vi "Scripting_GetStateMachineReferences_BaseReference.vi"(0 "Diagram":refnum<vi>, 1 "WhileLoop(False)":bool, 5 "error in (no error)":errorcluster) -> (12 "OutSideWhileLoopDiagram":refnum<vi>, 14 "StateMachine-WhileLoopDiagram":refnum<vi>, 15 "StateMachine-CaseSelector":refnum<vi>, 16 "Found":bool, 17 "Selector.Outside Terminal":refnum<vi>, 19 "error out":errorcluster)   [LabVIEW 2014]
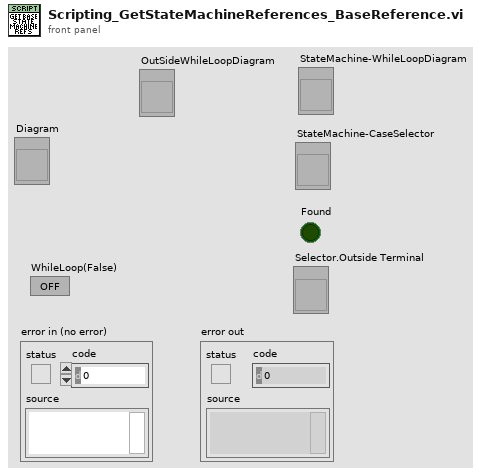
[diagram p1: front panel]
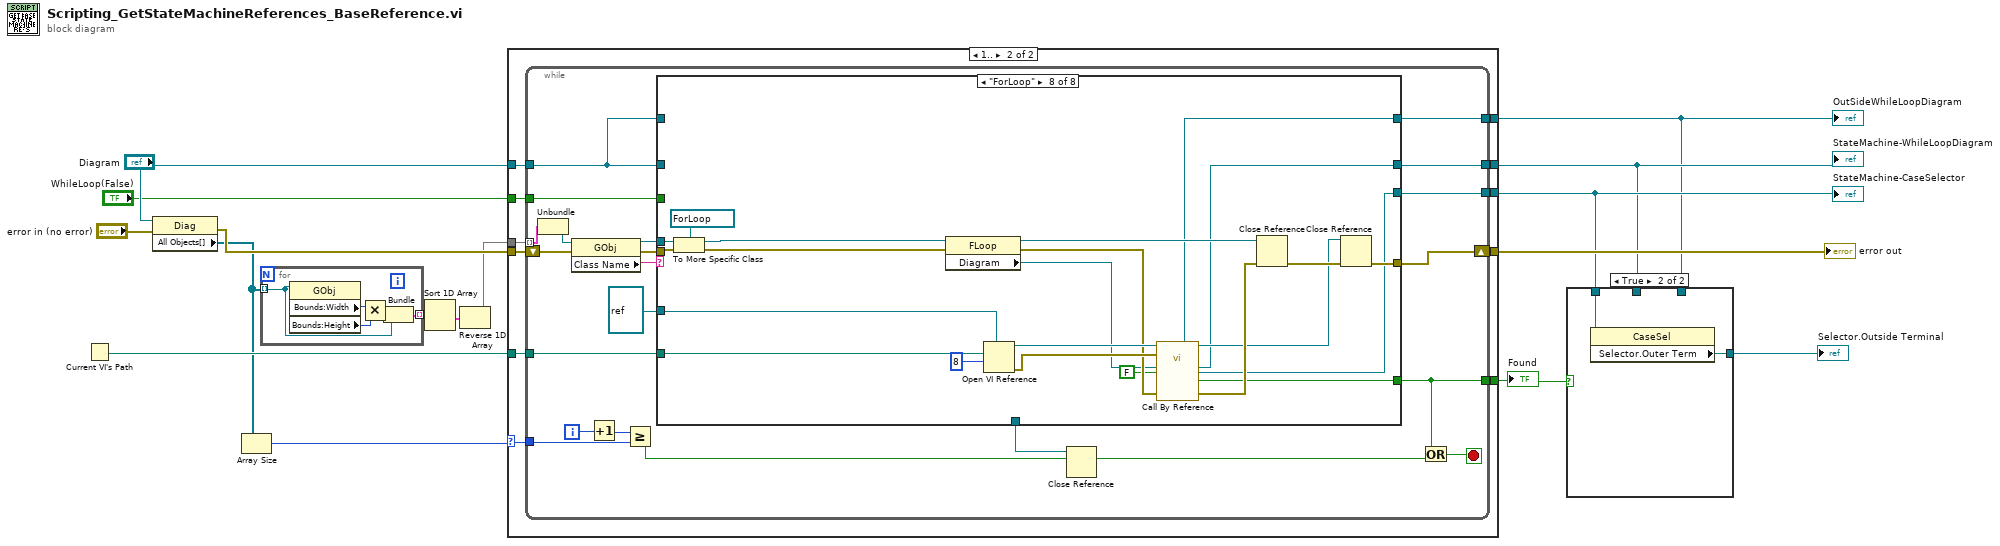
[diagram p0: block diagram]
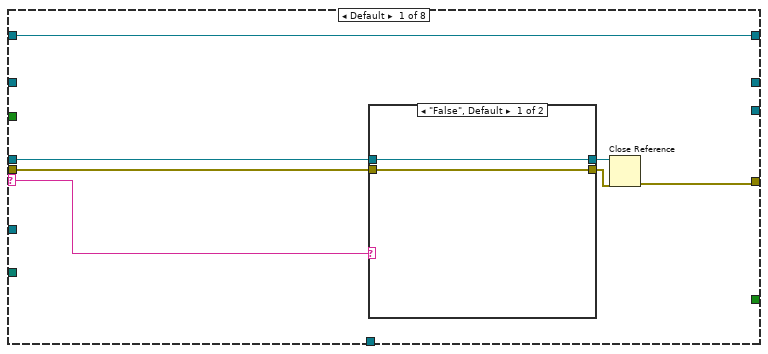
[diagram p3: hidden frame]
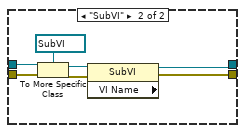
[diagram p4: hidden frame]
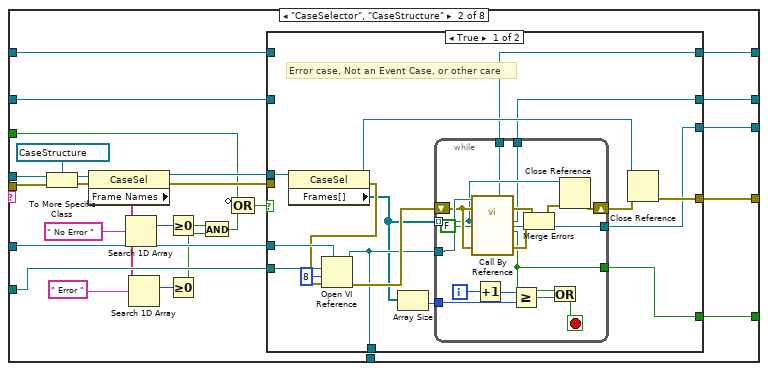
[diagram p5: hidden frame]
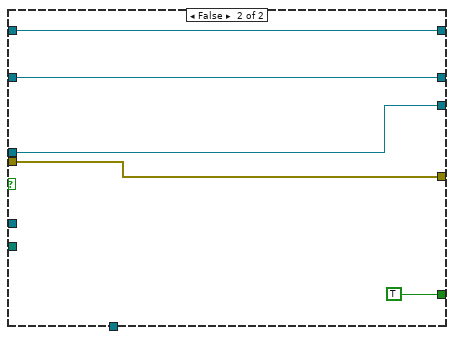
[diagram p6: hidden frame]
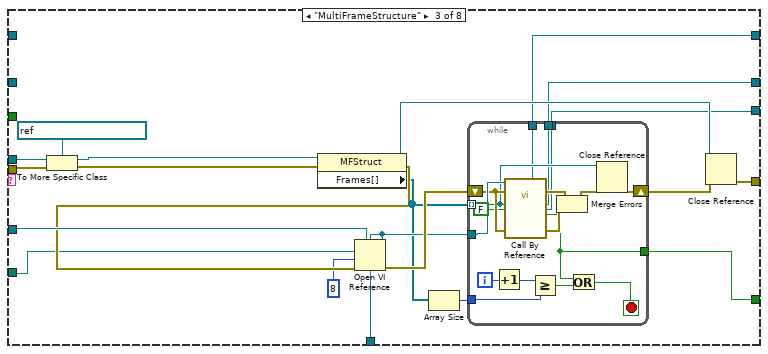
[diagram p7: hidden frame]
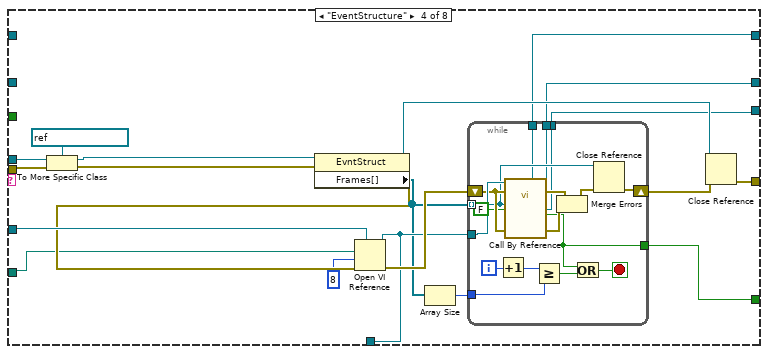
[diagram p8: hidden frame]
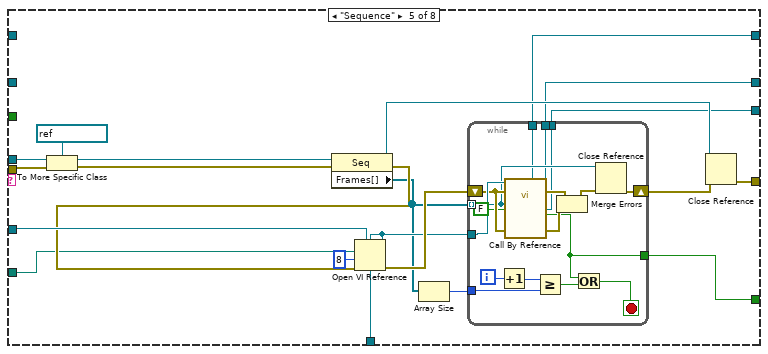
[diagram p9: hidden frame]
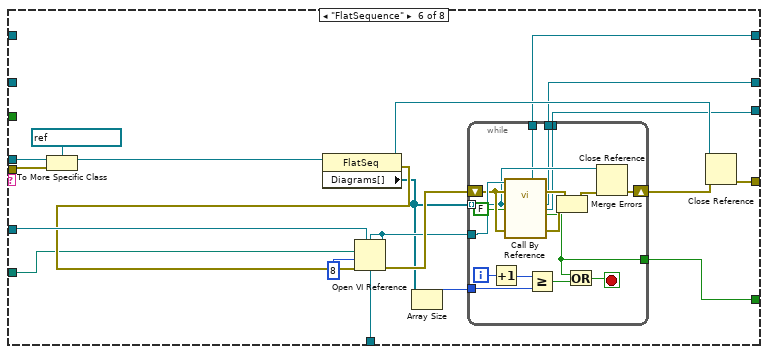
[diagram p10: hidden frame]
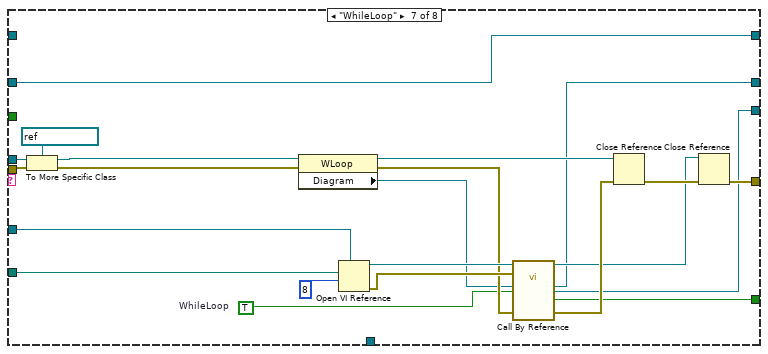
[diagram p11: hidden frame]
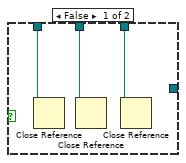
[diagram p12: hidden frame]
diagram:
  n1 = Current VI's Path() -> (path=w13:path)
  n2 = property class="Diag"(reference="Diagram", error in="error in (no error)") -> (error out=w15:errorcluster, "All Objects[]"=w3:refnum<vi>[])  [unwired: 1 out]
  n3 = Array Size(array=w3) -> (size(s)=w6:i32)
  n4 = for {
    tunnel: w3 -> [w17] mode=indexing
    tunnel: [w18] -> w5 mode=indexing
    n5 = property class="GObj"(reference=w17) -> ("Bounds:Width"=w21:u32, "Bounds:Height"=w20:u32)  [unwired: 1 in, 2 out]
    n6 = Multiply(x=w21, y=w20) -> (x*y=w19:u32)
    n7 = Bundle(w19, w17) -> (w18:cluster{u32, refnum<vi>})  [unwired: 1 out]
  }
  n8 = Sort 1D Array(array=w5) -> (sorted array=w4:cluster{u32, refnum<vi>}[])
  n9 = Reverse 1D Array(array=w4) -> (reversed array=w2:cluster{u32, refnum<vi>}[])
  n10 = case shown="1.." w6 {
    selector: w6 -> [_ w24]
    tunnel: w15 -> [w23 w34]
    tunnel: [w23 w33] -> w14
    tunnel: w13 -> [_ w32]
    tunnel: w2 -> [_ w31]
    tunnel: "Diagram" -> [w22 w30]
    tunnel: [_ w29] -> w11
    tunnel: [_ w28] -> w10
    tunnel: [_ w27] -> w9
    tunnel: [w22 w26] -> w8
    tunnel: "WhileLoop(False)" -> [_ w25]
    frame 0, Default {
    }
    frame 1.. {
      n11 = while {
        tunnel: w31 -> [w55] mode=indexing
        shift-right: [w50] -> w33
        shift-left: w34 -> [w52]
        tunnel: w32 -> [w48]
        tunnel: w24 -> [w44]
        tunnel: [w41] -> w28
        tunnel: [w40] -> w29
        tunnel: [w39] -> w26
        tunnel: [w38] -> w27
        tunnel: w30 -> [w37]
        tunnel: w25 -> [w36]
        i -> [w46]
        stop <- w42 stop-if-true
        n12 = Unbundle(w55) -> (w35:refnum<vi>)  [unwired: 1 out]
        n13 = property class="GObj"(reference=w35, error in=w52) -> (reference out=w53:refnum<vi>, error out=w51:errorcluster, "Class Name"=w54:string)
        n14 = Increment(x=w46) -> (x+1=w45:i32)
        n15 = Greater Or Equal?(x=w45, y=w44) -> (x >= y?=w43:bool)
        n16 = case shown="\"ForLoop\"" w54 {
          selector: w54 -> [w61 _ _ _ _ _ _ _]
          tunnel: w53 -> [w59 w98 w156 w193 w230 w266 w305 w327]
          tunnel: w51 -> [w60 w97 w153 w190 w227 w265 w299 w321]
          tunnel: [w62 w96 w152 w189 w226 w264 w292 w314] -> w50
          tunnel: refnum<vi> refnum ("VI Refnum") -> [_ w95 w149 w186 w223 w262 w294 w316]
          tunnel: w48 -> [_ w94 w145 w182 w220 w256 w290 w312]
          tunnel: [_ w93 w144 w181 w218 w255 _ _] -> w47
          tunnel: [_ w89 w140 w177 w216 w253 w288 w310] -> w40
          tunnel: [_ w88 w141 w178 w217 w254 w289 w311] -> w41
          tunnel: w37 -> [_ w83 _ _ _ _ w286 _]
          tunnel: [_ w82 w139 w176 w213 w250 w287 w309] -> w38
          tunnel: w37 -> [w56 w76 _ _ _ _ _ _]
          tunnel: [w56 w75 w138 w175 w212 w249 w286 w308] -> w39
          tunnel: w36 -> [_ w72 _ _ _ _ _ _]
          frame Default {
            n17 = case shown="\"False\", Default" w61 {
              tunnel: w60 -> [w64 w69]
              tunnel: w59 -> [w63 w70]
              tunnel: [w64 w67] -> w58
              tunnel: [w63 w66] -> w57
              frame "False", Default {
              }
              frame "SubVI" {
                n18 = To More Specific Class(target class=refnum<vi> refnum ("WhileLoop"), reference=w70, error in=w69) -> (specific class reference=w68:refnum<vi>, error out=w65:errorcluster)
                n19 = property class="SubVI" props=["VI Name"](reference=w68, error in=w65) -> (reference out=w66:refnum<vi>, error out=w67:errorcluster)  [unwired: 1 out]
              }
            }
            n20 = Close Reference(reference=w57, error in (no error)=w58) -> (error out=w62:errorcluster)
          }
          frame "CaseSelector", "CaseStructure" {
            n21 = To More Specific Class(target class=refnum<vi> refnum ("CaseSelector"), reference=w98, error in=w97) -> (specific class reference=w85:refnum<vi>, error out=w84:errorcluster)
            n22 = property class="CaseSel"(reference=w85, error in=w84) -> (reference out=w87:refnum<vi>, error out=w86:errorcluster, "Frame Names"=w81:string[])
            n23 = Search 1D Array(1D array=w81, element=" No Error ") -> (index of element=w90:i32)  [unwired: 1 in]
            n24 = Search 1D Array(1D array=w81, element=" Error ") -> (index of element=w78:i32)  [unwired: 1 in]
            n25 = Greater Or Equal To 0?(x=w90) -> (x >= 0?=w79:bool)
            n26 = Greater Or Equal To 0?(x=w78) -> (x >= 0?=w77:bool)
            n27 = And(x=w79, y=w77) -> (x .and. y?=w74:bool)
            n28 = Compound Arithmetic op=OR(invert w72, w74) -> (w73:bool)
            n29 = case shown="True" w73 {
              tunnel: [w114 w134] -> w96
              tunnel: w95 -> [w111 _]
              tunnel: w94 -> [w108 _]
              tunnel: [w107 _] -> w93
              tunnel: [w102 TRUE] -> w89
              tunnel: [w103 w135] -> w88
              tunnel: w87 -> [w106 w135]
              tunnel: w86 -> [_ w134]
              tunnel: w83 -> [_ w133]
              tunnel: [w101 w133] -> w82
              tunnel: w76 -> [_ w132]
              tunnel: [w100 w132] -> w75
              frame True {
                # "Error case, Not an Event Case, or other care"
                n30 = property class="CaseSel"(reference=w106) -> (reference out=w112:refnum<vi>, error out=w110:errorcluster, "Frames[]"=w105:refnum<vi>[])  [unwired: 1 in]
                n31 = Open VI Reference(type specifier VI Refnum (for type only)=w111, vi path=w108, options=8, error in (no error)=w110) -> (vi reference=w107:refnum<vi>, error out=w113:errorcluster)  [unwired: 2 out]
                n32 = Array Size(array=w105) -> (size(s)=w104:i32)
                n33 = while {
                  tunnel: w105 -> [w125] mode=indexing
                  shift-right: [w127] -> w109
                  shift-left: w113 -> [w129]
                  tunnel: w107 -> [w130]
                  tunnel: w104 -> [w122]
                  tunnel: [w119] -> w103
                  tunnel: [w118] -> w102
                  tunnel: [w117] -> w101
                  tunnel: [w116] -> w100
                  i -> [w123]
                  stop <- w121 stop-if-true
                  n34 = call-by-ref "?"(reference=w130, error in=w129, "Diagram"=w125, "WhileLoop(False)"=FALSE, "error in (no error)"=w129) -> (error out=w131:errorcluster, "OutSideWhileLoopDiagram"=w116:refnum<vi>, "StateMachine-WhileLoopDiagram"=w117:refnum<vi>, "StateMachine-CaseSelector"=w119:refnum<vi>, "Found"=w118:bool, 19:"error out"=w128:errorcluster)  [unwired: 11 in, 2 out]
                  n35 = Increment(x=w123) -> (x+1=w124:i32)
                  n36 = Greater Or Equal?(x=w124, y=w122) -> (x >= y?=w120:bool)
                  n37 = Merge Errors(w131, w128) -> (w126:errorcluster)
                  n38 = Or(x=w118, y=w120) -> (x .or. y?=w121:bool)
                  n39 = Close Reference(reference=w125, error in (no error)=w126) -> (error out=w127:errorcluster)
                }
                n40 = Close Reference(reference=w112, error in (no error)=w109) -> (error out=w114:errorcluster)
              }
              frame False {
              }
            }
          }
          frame "MultiFrameStructure" {
            n41 = To More Specific Class(target class=refnum<vi> refnum ("MultiFrameStructure"), reference=w156, error in=w153) -> (specific class reference=w155:refnum<vi>, error out=w154:errorcluster)
            n42 = property class="MFStruct"(reference=w155, error in=w154) -> (reference out=w150:refnum<vi>, error out=w148:errorcluster, "Frames[]"=w143:refnum<vi>[])
            n43 = Open VI Reference(type specifier VI Refnum (for type only)=w149, vi path=w145, options=8, error in (no error)=w148) -> (vi reference=w144:refnum<vi>, error out=w151:errorcluster)  [unwired: 2 out]
            n44 = Array Size(array=w143) -> (size(s)=w142:i32)
            n45 = while {
              tunnel: w143 -> [w169] mode=indexing
              shift-right: [w167] -> w147
              shift-left: w151 -> [w171]
              tunnel: w144 -> [w172]
              tunnel: w142 -> [w163]
              tunnel: [w161] -> w141
              tunnel: [w160] -> w140
              tunnel: [w159] -> w139
              tunnel: [w158] -> w138
              i -> [w164]
              stop <- w162 stop-if-true
              n46 = Increment(x=w164) -> (x+1=w166:i32)
              n47 = call-by-ref "?"(reference=w172, error in=w171, "Diagram"=w169, "WhileLoop(False)"=FALSE, "error in (no error)"=w171) -> (error out=w173:errorcluster, "OutSideWhileLoopDiagram"=w158:refnum<vi>, "StateMachine-WhileLoopDiagram"=w159:refnum<vi>, "StateMachine-CaseSelector"=w161:refnum<vi>, "Found"=w160:bool, 19:"error out"=w170:errorcluster)  [unwired: 11 in, 2 out]
              n48 = Greater Or Equal?(x=w166, y=w163) -> (x >= y?=w165:bool)
              n49 = Merge Errors(w173, w170) -> (w168:errorcluster)
              n50 = Or(x=w160, y=w165) -> (x .or. y?=w162:bool)
              n51 = Close Reference(reference=w169, error in (no error)=w168) -> (error out=w167:errorcluster)
            }
            n52 = Close Reference(reference=w150, error in (no error)=w147) -> (error out=w152:errorcluster)
          }
          frame "EventStructure" {
            n53 = To More Specific Class(target class=refnum<vi> refnum ("EventStructure"), reference=w193, error in=w190) -> (specific class reference=w192:refnum<vi>, error out=w191:errorcluster)
            n54 = property class="EvntStruct"(reference=w192, error in=w191) -> (reference out=w187:refnum<vi>, error out=w185:errorcluster, "Frames[]"=w180:refnum<vi>[])
            n55 = Open VI Reference(type specifier VI Refnum (for type only)=w186, vi path=w182, options=8, error in (no error)=w185) -> (vi reference=w181:refnum<vi>, error out=w188:errorcluster)  [unwired: 2 out]
            n56 = Array Size(array=w180) -> (size(s)=w179:i32)
            n57 = while {
              tunnel: w180 -> [w204] mode=indexing
              shift-right: [w205] -> w184
              shift-left: w188 -> [w208]
              tunnel: w181 -> [w209]
              tunnel: w179 -> [w200]
              tunnel: [w199] -> w178
              tunnel: [w198] -> w177
              tunnel: [w196] -> w176
              tunnel: [w195] -> w175
              i -> [w201]
              stop <- w197 stop-if-true
              n58 = Increment(x=w201) -> (x+1=w203:i32)
              n59 = call-by-ref "?"(reference=w209, error in=w208, "Diagram"=w204, "WhileLoop(False)"=FALSE, "error in (no error)"=w208) -> (error out=w210:errorcluster, "OutSideWhileLoopDiagram"=w195:refnum<vi>, "StateMachine-WhileLoopDiagram"=w196:refnum<vi>, "StateMachine-CaseSelector"=w199:refnum<vi>, "Found"=w198:bool, 19:"error out"=w207:errorcluster)  [unwired: 11 in, 2 out]
              n60 = Greater Or Equal?(x=w203, y=w200) -> (x >= y?=w202:bool)
              n61 = Merge Errors(w210, w207) -> (w206:errorcluster)
              n62 = Or(x=w198, y=w202) -> (x .or. y?=w197:bool)
              n63 = Close Reference(reference=w204, error in (no error)=w206) -> (error out=w205:errorcluster)
            }
            n64 = Close Reference(reference=w187, error in (no error)=w184) -> (error out=w189:errorcluster)
          }
          frame "Sequence" {
            n65 = To More Specific Class(target class=refnum<vi> refnum ("Sequence"), reference=w230, error in=w227) -> (specific class reference=w229:refnum<vi>, error out=w228:errorcluster)
            n66 = property class="Seq"(reference=w229, error in=w228) -> (reference out=w224:refnum<vi>, error out=w222:errorcluster, "Frames[]"=w215:refnum<vi>[])
            n67 = Open VI Reference(type specifier VI Refnum (for type only)=w223, vi path=w220, options=8, error in (no error)=w222) -> (vi reference=w218:refnum<vi>, error out=w225:errorcluster)  [unwired: 2 out]
            n68 = Array Size(array=w215) -> (size(s)=w214:i32)
            n69 = while {
              tunnel: w215 -> [w241] mode=indexing
              shift-right: [w243] -> w219
              shift-left: w225 -> [w245]
              tunnel: w218 -> [w246]
              tunnel: [w236] -> w217
              tunnel: [w235] -> w216
              tunnel: w214 -> [w234]
              tunnel: [w233] -> w213
              tunnel: [w232] -> w212
              i -> [w238]
              stop <- w237 stop-if-true
              n70 = Increment(x=w238) -> (x+1=w240:i32)
              n71 = call-by-ref "?"(reference=w246, error in=w245, "Diagram"=w241, "WhileLoop(False)"=FALSE, "error in (no error)"=w245) -> (error out=w247:errorcluster, "OutSideWhileLoopDiagram"=w232:refnum<vi>, "StateMachine-WhileLoopDiagram"=w233:refnum<vi>, "StateMachine-CaseSelector"=w236:refnum<vi>, "Found"=w235:bool, 19:"error out"=w244:errorcluster)  [unwired: 11 in, 2 out]
              n72 = Greater Or Equal?(x=w240, y=w234) -> (x >= y?=w239:bool)
              n73 = Merge Errors(w247, w244) -> (w242:errorcluster)
              n74 = Or(x=w235, y=w239) -> (x .or. y?=w237:bool)
              n75 = Close Reference(reference=w241, error in (no error)=w242) -> (error out=w243:errorcluster)
            }
            n76 = Close Reference(reference=w224, error in (no error)=w219) -> (error out=w226:errorcluster)
          }
          frame "FlatSequence" {
            n77 = To More Specific Class(target class=refnum<vi> refnum ("FlatSequence"), reference=w266, error in=w265) -> (specific class reference=w259:refnum<vi>)  [unwired: 1 out]
            n78 = property class="FlatSeq"(reference=w259) -> (reference out=w257:refnum<vi>, error out=w258:errorcluster, "Diagrams[]"=w252:refnum<vi>[])  [unwired: 1 in]
            n79 = Open VI Reference(type specifier VI Refnum (for type only)=w262, vi path=w256, options=8, error in (no error)=w258) -> (vi reference=w255:refnum<vi>, error out=w263:errorcluster)  [unwired: 2 out]
            n80 = Array Size(array=w252) -> (size(s)=w251:i32)
            n81 = while {
              tunnel: w252 -> [w277] mode=indexing
              shift-right: [w279] -> w261
              shift-left: w263 -> [w281]
              tunnel: w255 -> [w282]
              tunnel: [w272] -> w254
              tunnel: [w271] -> w253
              tunnel: w251 -> [w270]
              tunnel: [w269] -> w250
              tunnel: [w268] -> w249
              i -> [w274]
              stop <- w273 stop-if-true
              n82 = Increment(x=w274) -> (x+1=w276:i32)
              n83 = call-by-ref "?"(reference=w282, error in=w281, "Diagram"=w277, "WhileLoop(False)"=FALSE, "error in (no error)"=w281) -> (error out=w283:errorcluster, "OutSideWhileLoopDiagram"=w268:refnum<vi>, "StateMachine-WhileLoopDiagram"=w269:refnum<vi>, "StateMachine-CaseSelector"=w272:refnum<vi>, "Found"=w271:bool, 19:"error out"=w280:errorcluster)  [unwired: 11 in, 2 out]
              n84 = Greater Or Equal?(x=w276, y=w270) -> (x >= y?=w275:bool)
              n85 = Merge Errors(w283, w280) -> (w278:errorcluster)
              n86 = Or(x=w271, y=w275) -> (x .or. y?=w273:bool)
              n87 = Close Reference(reference=w277, error in (no error)=w278) -> (error out=w279:errorcluster)
            }
            n88 = Close Reference(reference=w257, error in (no error)=w261) -> (error out=w264:errorcluster)
          }
          frame "WhileLoop" {
            w285 = TRUE  # WhileLoop
            n89 = To More Specific Class(target class=refnum<vi> refnum ("WhileLoop"), reference=w305, error in=w299) -> (specific class reference=w304:refnum<vi>, error out=w300:errorcluster)
            n90 = property class="WLoop"(reference=w304, error in=w300) -> (reference out=w302:refnum<vi>, error out=w296:errorcluster, "Diagram"=w295:refnum<vi>)
            n91 = Open VI Reference(type specifier VI Refnum (for type only)=w294, vi path=w290, options=8) -> (vi reference=w298:refnum<vi>, error out=w301:errorcluster)  [unwired: 1 in, 2 out]
            n92 = call-by-ref "?"(reference=w298, error in=w301, "Diagram"=w295, "WhileLoop(False)"=w285, "error in (no error)"=w296) -> (reference out=w291:refnum<vi>, "StateMachine-WhileLoopDiagram"=w287:refnum<vi>, "StateMachine-CaseSelector"=w289:refnum<vi>, "Found"=w288:bool, "error out"=w297:errorcluster)  [unwired: 11 in, 3 out]
            n93 = Close Reference(reference=w302, error in (no error)=w297) -> (error out=w293:errorcluster)
            n94 = Close Reference(reference=w291, error in (no error)=w293) -> (error out=w292:errorcluster)
          }
          frame "ForLoop" {
            n95 = To More Specific Class(target class=refnum<vi> refnum ("WhileLoop"), reference=w327, error in=w321) -> (specific class reference=w326:refnum<vi>, error out=w322:errorcluster)
            n96 = property class="FLoop"(reference=w326, error in=w322) -> (reference out=w324:refnum<vi>, error out=w318:errorcluster, "Diagram"=w317:refnum<vi>)
            n97 = Open VI Reference(type specifier VI Refnum (for type only)=w316, vi path=w312, options=8) -> (vi reference=w320:refnum<vi>, error out=w323:errorcluster)  [unwired: 1 in, 2 out]
            n98 = call-by-ref "?"(reference=w320, error in=w323, "Diagram"=w317, "WhileLoop(False)"=FALSE, "error in (no error)"=w318) -> (reference out=w313:refnum<vi>, "OutSideWhileLoopDiagram"=w308:refnum<vi>, "StateMachine-WhileLoopDiagram"=w309:refnum<vi>, "StateMachine-CaseSelector"=w311:refnum<vi>, "Found"=w310:bool, "error out"=w319:errorcluster)  [unwired: 11 in, 2 out]
            n99 = Close Reference(reference=w324, error in (no error)=w319) -> (error out=w315:errorcluster)
            n100 = Close Reference(reference=w313, error in (no error)=w315) -> (error out=w314:errorcluster)
          }
        }
        n101 = Close Reference(reference=w47) -> ()  [unwired: 1 in, 1 out]
        n102 = Or(x=w40, y=w43) -> (x .or. y?=w42:bool)
      }
    }
  }
  "error out" <- w14
  "StateMachine-CaseSelector" <- w10
  "Found" <- w11
  "StateMachine-WhileLoopDiagram" <- w9
  "OutSideWhileLoopDiagram" <- w8
  n103 = case shown="True" w11 {
    tunnel: w10 -> [w330 w332]
    tunnel: w9 -> [w329 _]
    tunnel: w8 -> [w328 _]
    tunnel: [_ w331] -> w1
    frame False {
      n104 = Close Reference(reference=w330) -> ()  [unwired: 1 in, 1 out]
      n105 = Close Reference(reference=w329) -> ()  [unwired: 1 in, 1 out]
      n106 = Close Reference(reference=w328) -> ()  [unwired: 1 in, 1 out]
    }
    frame True {
      n107 = property class="CaseSel"(reference=w332) -> ("Selector.Outer Term"=w331:refnum<vi>)  [unwired: 1 in, 2 out]
    }
  }
  "Selector.Outside Terminal" <- w1
